vi "Initialize.vi"(8 "error in (no error)":errorcluster, 9 "Reset (True)":bool=TRUE, 10 "ID Query (True)":bool=TRUE, 11 "VISA resource name":refnum<visa-resource-name>="USB0::0x2A8D::0x7F18::MY58240013::INSTR") -> (0 "error out":errorcluster, 3 "VISA resource name out":refnum<visa-resource-name>="USB0::0x2A8D::0x7F18::MY58240013::INSTR", 5 "IDN?(str)":string="U2022XA,MY58240013,A.04.06\n", 7 "Success?(t)":bool)   [LabVIEW 2018, in "Agilent U2000 Series.lvlib"]
doc: "Establishes communication with the instrument and optionally performs an instrument identification query and/or an instrument reset. It also places the instrument in a default state needed for other instrument driver operations. Therefore, call this VI before calling other instrument driver VIs for this instrument. Generally, you need to call the Initialize VI only once at the beginning of an application."
uses:
  Agilent U2000 Series.lvlib
  Private/Extended User Data.ctl
  <vilib>/regexp/Match Regular Expression.xnode
panel:
  # "(c) 2011-2015 National Instruments.  ALL RIGHTS RESERVED."
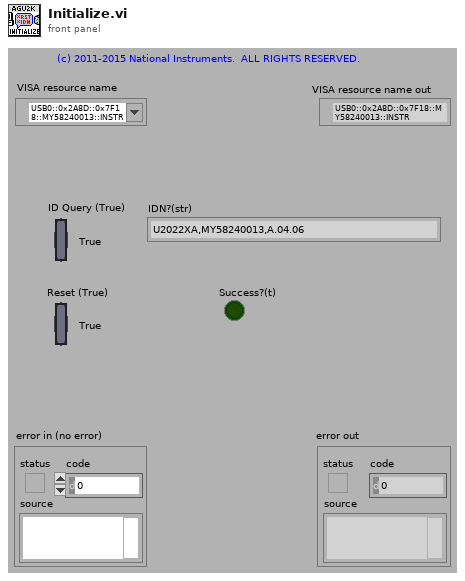
[diagram p1: front panel]
types:
  T1 = typedef "Agilent U2000 Series.lvlib/Extended User Data.ctl" = cluster{"U2000 Series Mode":u16, "Trigger Source Int/Ext":bool}
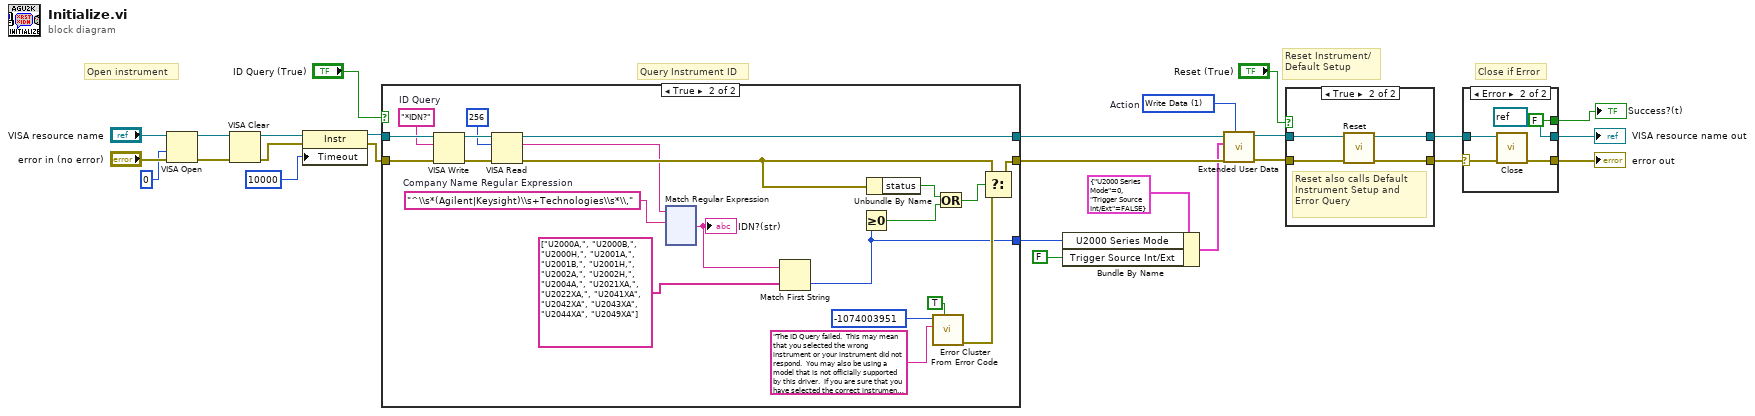
[diagram p0: block diagram]
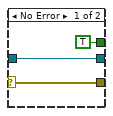
[diagram p2: hidden frame]
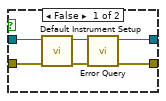
[diagram p3: hidden frame]
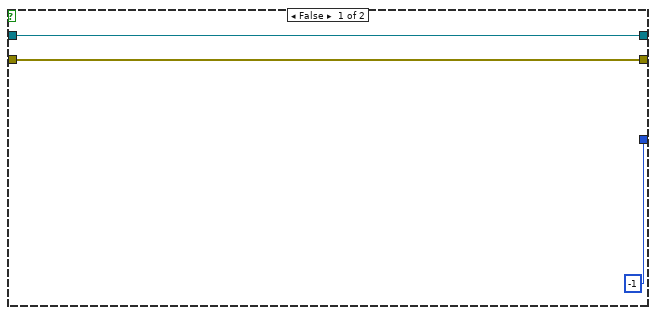
[diagram p4: hidden frame]
diagram:
  w6 = 1 items=["Read Data", "Write Data", "Clear Data", "Clear ALL Data"]  # Action
  # "Close if Error"
  # "Query Instrument ID"
  # "Reset Instrument/\nDefault Setup"
  # "Open instrument"
  n1 = VISA Open(access mode=u32 0, error in (no error)="error in (no error)", VISA resource name="VISA resource name") -> (VISA resource name=w21:refnum<visa-resource-name>, error out=w20:errorcluster)  [unwired: 2 out]
  n2 = VISA Clear(VISA resource name=w21, error in (no error)=w20) -> (VISA resource name out=w15:refnum<visa-resource-name>, error out=w14:errorcluster)
  n3 = property class="Instr"(reference=w15, error in=w14, "Timeout"=u32 10000 ("General Settings:Timeout Value")) -> (reference out=w12:refnum<visa-resource-name>, error out=w11:errorcluster)
  n4 = case shown="True" "ID Query (True)" {
    tunnel: [w28 w50] -> w7
    tunnel: [w29 w47] -> w8
    tunnel: w12 -> [w29 w48]
    tunnel: w11 -> [w28 w49]
    tunnel: [-1 ("index") w33] -> w5
    frame False {
    }
    frame True {
      w30 = "^\\s*(Agilent|Keysight)\\s+Technologies\\s*\\,"  # Company Name Regular Expression
      w43 = "*IDN?"  # ID Query
      n5 = VISA Write(VISA resource name=w48, write buffer=w43, error in (no error)=w49) -> (VISA resource name out=w46:refnum<visa-resource-name>, error out=w45:errorcluster)  [unwired: 1 out]
      n6 = VISA Read(VISA resource name=w46, byte count=u32 256, error in (no error)=w45) -> (VISA resource name out=w47:refnum<visa-resource-name>, read buffer=w32:string, error out=w38:errorcluster)  [unwired: 1 out]
      n7 = xnode "Match Regular Expression"("input string"=w32, "regular expression"=w30) -> ("after match"=w31:string)  [unwired: 4 in, 4 out]
      "IDN?(str)" <- w31
      n8 = Match First String(2:string[] ["U2000A,", "U2000B,", "U2000H,", "U2001A,", "U2001B,", "U2001H,", "U2002A,", "U2002H,", "U2004A,", "U2021XA,", "U2022XA,", "U2041XA", "U2042XA", "U2043XA", "U2044XA", "U2049XA"] ("string array"), 3:w31) -> (0:w33:i32)  [unwired: 1 out]
      n9 = Greater Or Equal To 0?(x=w33) -> (x >= 0?=w36:bool)
      n10 = Unbundle By Name(w38) -> ("status"=w37:bool)
      n11 = call <vilib>:"Error Cluster From Error Code.vi"("show call chain? (False)"=TRUE, "error message (\"\")"="The ID Query failed.  This may mean that you selected the wrong instrument or your instrument did not respond.  You may also be using a model that is not officially supported by this driver.  If you are sure that you have selected the correct instrument and it is responding, try disabling the ID Query." ("Source (VI Name)"), "error code (0)"=-1074003951 ("Code")) -> ("error out"=w42:errorcluster)  [unwired: 1 in, 5 out]
      n12 = Or(x=w37, y=w36) -> (x .or. y?=w35:bool)
      n13 = Select(t=w38, s=w35, f=w42) -> (s? t:f=w50:errorcluster)
    }
  }
  n14 = Bundle By Name(cluster=T1 {"U2000 Series Mode"=0, "Trigger Source Int/Ext"=FALSE} ("output cluster"), "U2000 Series Mode"=w5, "Trigger Source Int/Ext"=FALSE) -> (w3:T1)
  n15 = call "Extended User Data.vi"("Action (1: Write Data)"=w6, "error in (no error)"=w7, "User Data In"=w3, "VISA resource name"=w8) -> ("error out"=w9:errorcluster, "VISA resource name out"=w10:refnum<visa-resource-name>)  [unwired: 6 out]
  n16 = case shown="True" "Reset (True)" {
    tunnel: w9 -> [w169 w171]
    tunnel: [w166 w174] -> w16
    tunnel: w10 -> [w170 w172]
    tunnel: [w167 w173] -> w17
    frame False {
      n17 = call "Default Instrument Setup.vi"("error in (no error)"=w169, "VISA resource name"=w170) -> ("error out"=w165:errorcluster, "VISA resource name out"=w168:refnum<visa-resource-name>)  [unwired: 8 out]
      n18 = call "Error Query.vi"("error in (no error)"=w165, "VISA resource name"=w168) -> ("error out"=w166:errorcluster, "VISA resource name out"=w167:refnum<visa-resource-name>)  [unwired: 8 out]
    }
    frame True {
      # "Reset also calls Default Instrument Setup and Error Query"
      n19 = call "Reset.vi"("error in (no error)"=w171, "VISA resource name"=w172) -> ("error out"=w174:errorcluster, "VISA resource name out"=w173:refnum<visa-resource-name>)  [unwired: 8 out]
    }
  }
  n20 = case shown="Error" w16 {
    selector: w16 -> [w176 w180]
    tunnel: w17 -> [w177 w181]
    tunnel: [w177 refnum<visa-resource-name> refnum ("VISA resource name out")] -> w19
    tunnel: [w176 w182] -> w18
    tunnel: [TRUE ("Success?(t)") FALSE ("Success?(t)")] -> w1
    frame No Error {
    }
    frame Error {
      n21 = call "Close.vi"("error in (no error)"=w180, "VISA resource name"=w181) -> ("error out"=w182:errorcluster)  [unwired: 9 out]
    }
  }
  "VISA resource name out" <- w19
  "error out" <- w18
  "Success?(t)" <- w1
